vi "Player Info.vi"(8 "Victory Speech":string="What a tasty treat was this universe", 9 "Name":string="Expand", 11 "Expand in":refnum<class "Expand.lvclass">) -> (3 "Expand out":refnum<class "Expand.lvclass">)   [LabVIEW 2015, in "Expand.lvclass"]
uses:
  Expand.lvclass
  Square/Square.lvclass/Square.ctl
  Square/Write Name.vi
  Square/Write Victory Speech.vi
panel:
  # "Set default values for these two string controls"
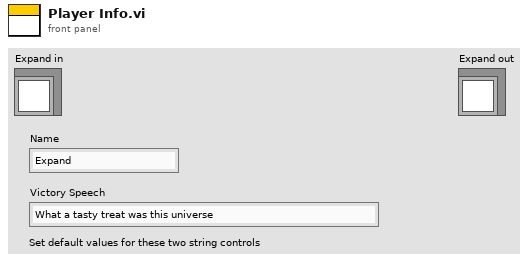
[diagram p1: front panel]
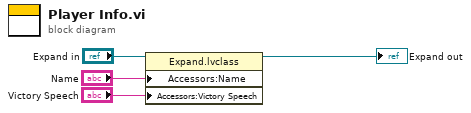
[diagram p0: block diagram]
diagram:
  n1 = property class="Expand.lvclass"(reference="Expand in", "Accessors:Name"="Name", "Accessors:Victory Speech"="Victory Speech") -> (reference out=→"Expand out":refnum<class "Expand.lvclass">)  [unwired: 1 in, 1 out]
